vi "Autonomous Independent.vi"() -> ()   [LabVIEW 2013]
doc: "This VI is called when autonomous begins, and will automatically be terminated when autonomous ends. You can carry out timed or sensor driven robot movement independently without needing to return to the caller."
uses:
  Program Files (x86)/National Instruments/LabVIEW 2013/examples/FRC/I2C/ADXL345 I2C/Driver/ADXL345 I2C Axis.ctl
  Robot Global Data.vi
  <vilib>/addons/control/pid/pid.llb/PID (DBL).vi
  <vilib>/Rock Robotics/WPI/RobotDrive/WPI_RobotDriveGetSetRefNum.vi
  <vilib>/Rock Robotics/WPI/Joystick/WPI_JoystickGetSetRefNum.vi
  <vilib>/Rock Robotics/WPI/RobotDrive/WPI_RobotDriveArcadeDrive_Standard(NoSaturation).vi
  <vilib>/addons/control/pid/NI_PID_pid.lvlib
panel:
  in  "PID gains":T1={"proportional gain (Kc)"=1.0, "integral time (Ti, min)"=0.01, "derivative time (Td, min)"=0.0} {"derivative time (Td, min)" format="%.3f"; "integral time (Ti, min)" format="%.3f"; "proportional gain (Kc)" format="%.3f"}
  in  "Stop":bool
  in  "SP:":dbl(slide)=60.7843137254902 min=0.0 max=0.0 scale=0.0..100.0
  out "MV:":dbl(slide)=18.78965245852964 scale=-100.0..100.0
  out "Current Movement, for debugging":T2 {"Y Joystick Value" scale=1.0..-1.0; "X Joystick Value" scale=-1.0..1.0}
  in  "Array of robot movements":T3(array[cluster]) {"Y Joystick Value" scale=1.0..-1.0; "X Joystick Value" scale=-1.0..1.0}
  # "Be sure to right-click and choose Data Operations>>Make Current Value default if you want to save the array values with the VI"
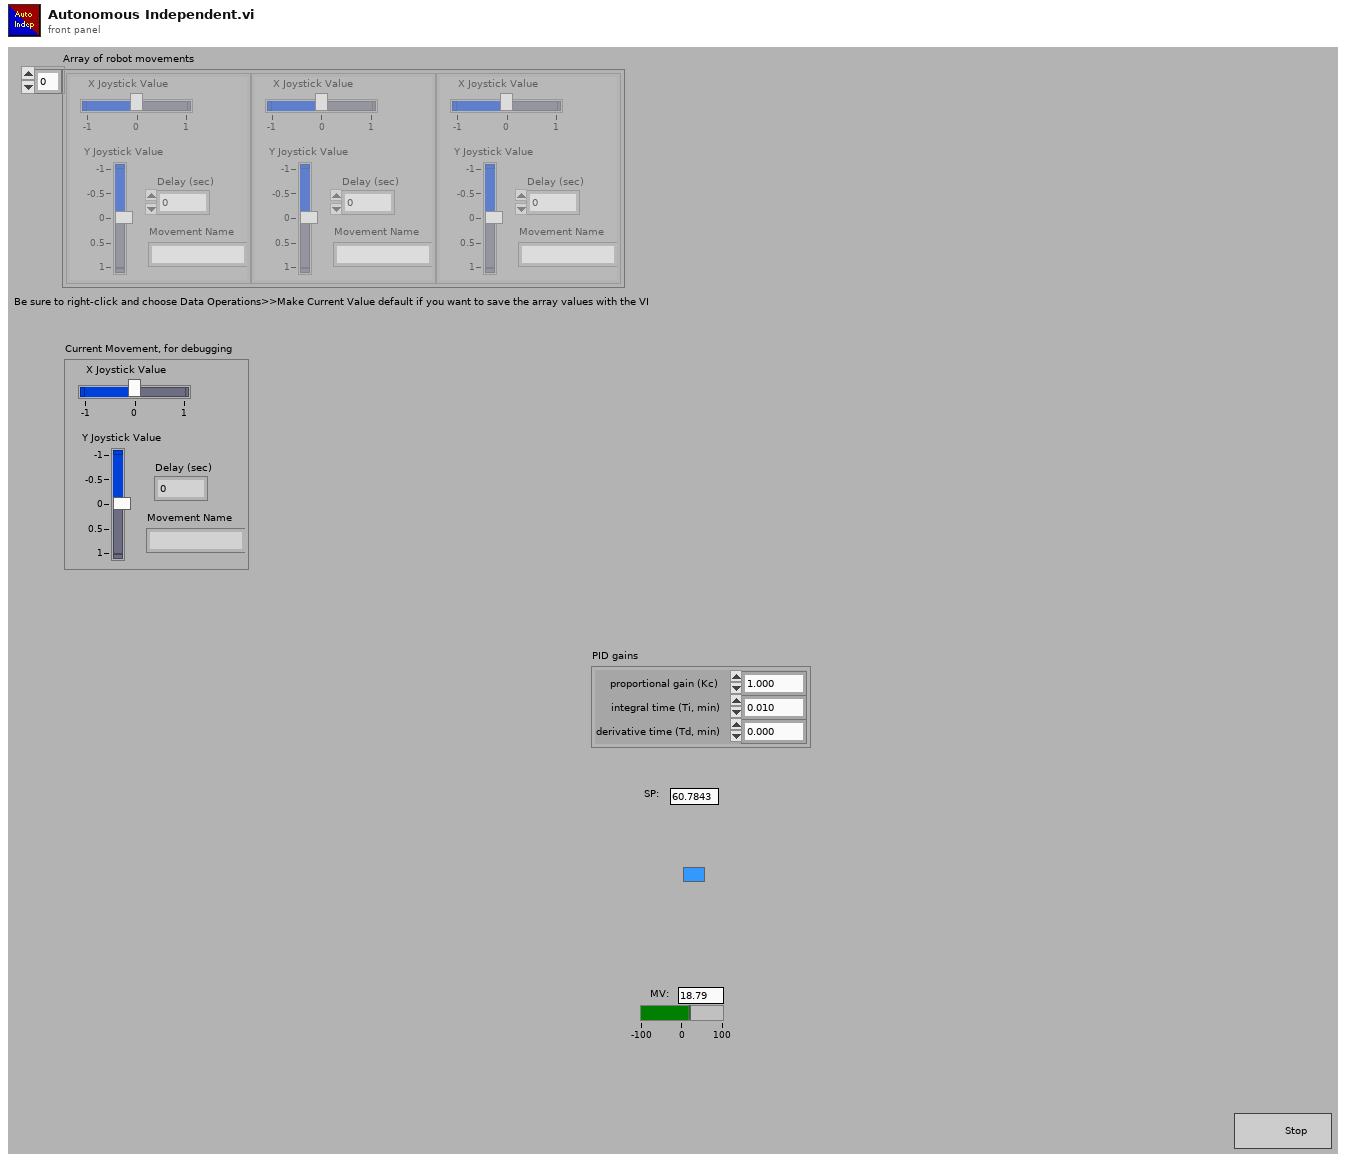
[diagram p1: front panel]
types:
  T1 = cluster{"proportional gain (Kc)":dbl, "integral time (Ti, min)":dbl, "derivative time (Td, min)":dbl}
  T2 = cluster{"X Joystick Value":dbl, "Y Joystick Value":dbl, "Delay (sec)":dbl, "Movement Name":string}
  T3 = cluster{"X Joystick Value":dbl, "Y Joystick Value":dbl, "Delay (sec)":dbl, "Movement Name":string}[]
  T4 = typedef "WPI_JoystickDevRef.ctl" = cluster{"Device":T5}
  T5 = typedef "WPI_JoystickDeviceEnum.ctl" = enum16{"USB 1", "USB 2", "USB 3", "USB 4", "Kinect 1", "Kinect 2"}
  T6 = typedef "WPI_EncoderDevRef.ctl" = cluster{"DevStatus":errorcluster, "EncoderIndex":T7, "CounterIndex":T8, "DistancePerCount":dbl, "Decoding Type":T9}
  T7 = typedef "FPGA_EncoderIdx.ctl" = enum8{"Enc 0", "Enc 1", "Enc 2", "Enc 3", "Invalid"}
  T8 = typedef "FPGA_CounterCtrSystemIndex.ctl" = enum8{"Ctr 0", "Ctr 1", "Ctr 2", "Ctr 3", "Ctr 4", "Ctr 5", "Ctr 6", "Ctr 7", "Invalid"}
  T9 = typedef "WPI_EncoderType.ctl" = enum16{"1x", "2x", "4x"}
  T10 = cluster{"axis 1 (x)":dbl, "axis 2 (y)":dbl, "axis 3 (throttle)":dbl, "axis 4":dbl, "axis 5":dbl, "axis 6":dbl}
  T11 = typedef "WPI_I2CDevRef.ctl" = cluster{"DevStatus":errorcluster, "Digital Module":T12, "Device Address":u8}
  T12 = typedef "FPGA_TypedefDigitalModule.ctl" = enum16{"Digital Module 1", "Digital Module 2"}
  T13 = typedef "WPI_RobotDriveDevRef.ctl" = cluster{"DevStatus":errorcluster, "Motors[]":T14[], "Square Inputs":bool, "Max Output":dbl, "Isochronous":bool}
  T14 = typedef "WPI_MotorControlDeviceRef.ctl" = cluster{"DeviceStatus":errorcluster, "Type":enum16{"PWM", "CAN"}, "PWM":cluster{"Digital Module":T12, "PWM Channel":T15, "DeadBand":T16}, "CAN":cluster{"Device Number":u8, "Control Mode":T17, "Semaphore":T18, "Max Vout":dbl}, "Invert":bool, "TransformRef":T19, "InvTransformRef":T19}
  T15 = typedef "FPGA_DIOPWMChannel.ctl" = enum8{"PWM 1", "PWM 2", "PWM 3", "PWM 4", "PWM 5", "PWM 6", "PWM 7", "PWM 8", "PWM 9", "PWM 10", "Invalid"}
  T16 = typedef "WPI_PWMDeadband.ctl" = cluster{"Name":string, "maxPositivePwm":i32, "minPositivePwm":i32, "centerPwm":i32, "maxNegativePwm":i32, "minNegativePwm":i32, "angularRange":u16}
  T17 = typedef "WPI_CANJaguar_ControlMode.ctl" = enum8{"Percent VBus", "Current", "Speed", "Position", "Voltage"}
  T18 = typedef "Semaphore RefNum" = refnum<k1>
  T19 = typedef "WPI_PWMTransform_ConPane.ctl" = refnum<vi>
  T20 = typedef "ADXL345 I2C Axis.ctl" = u8
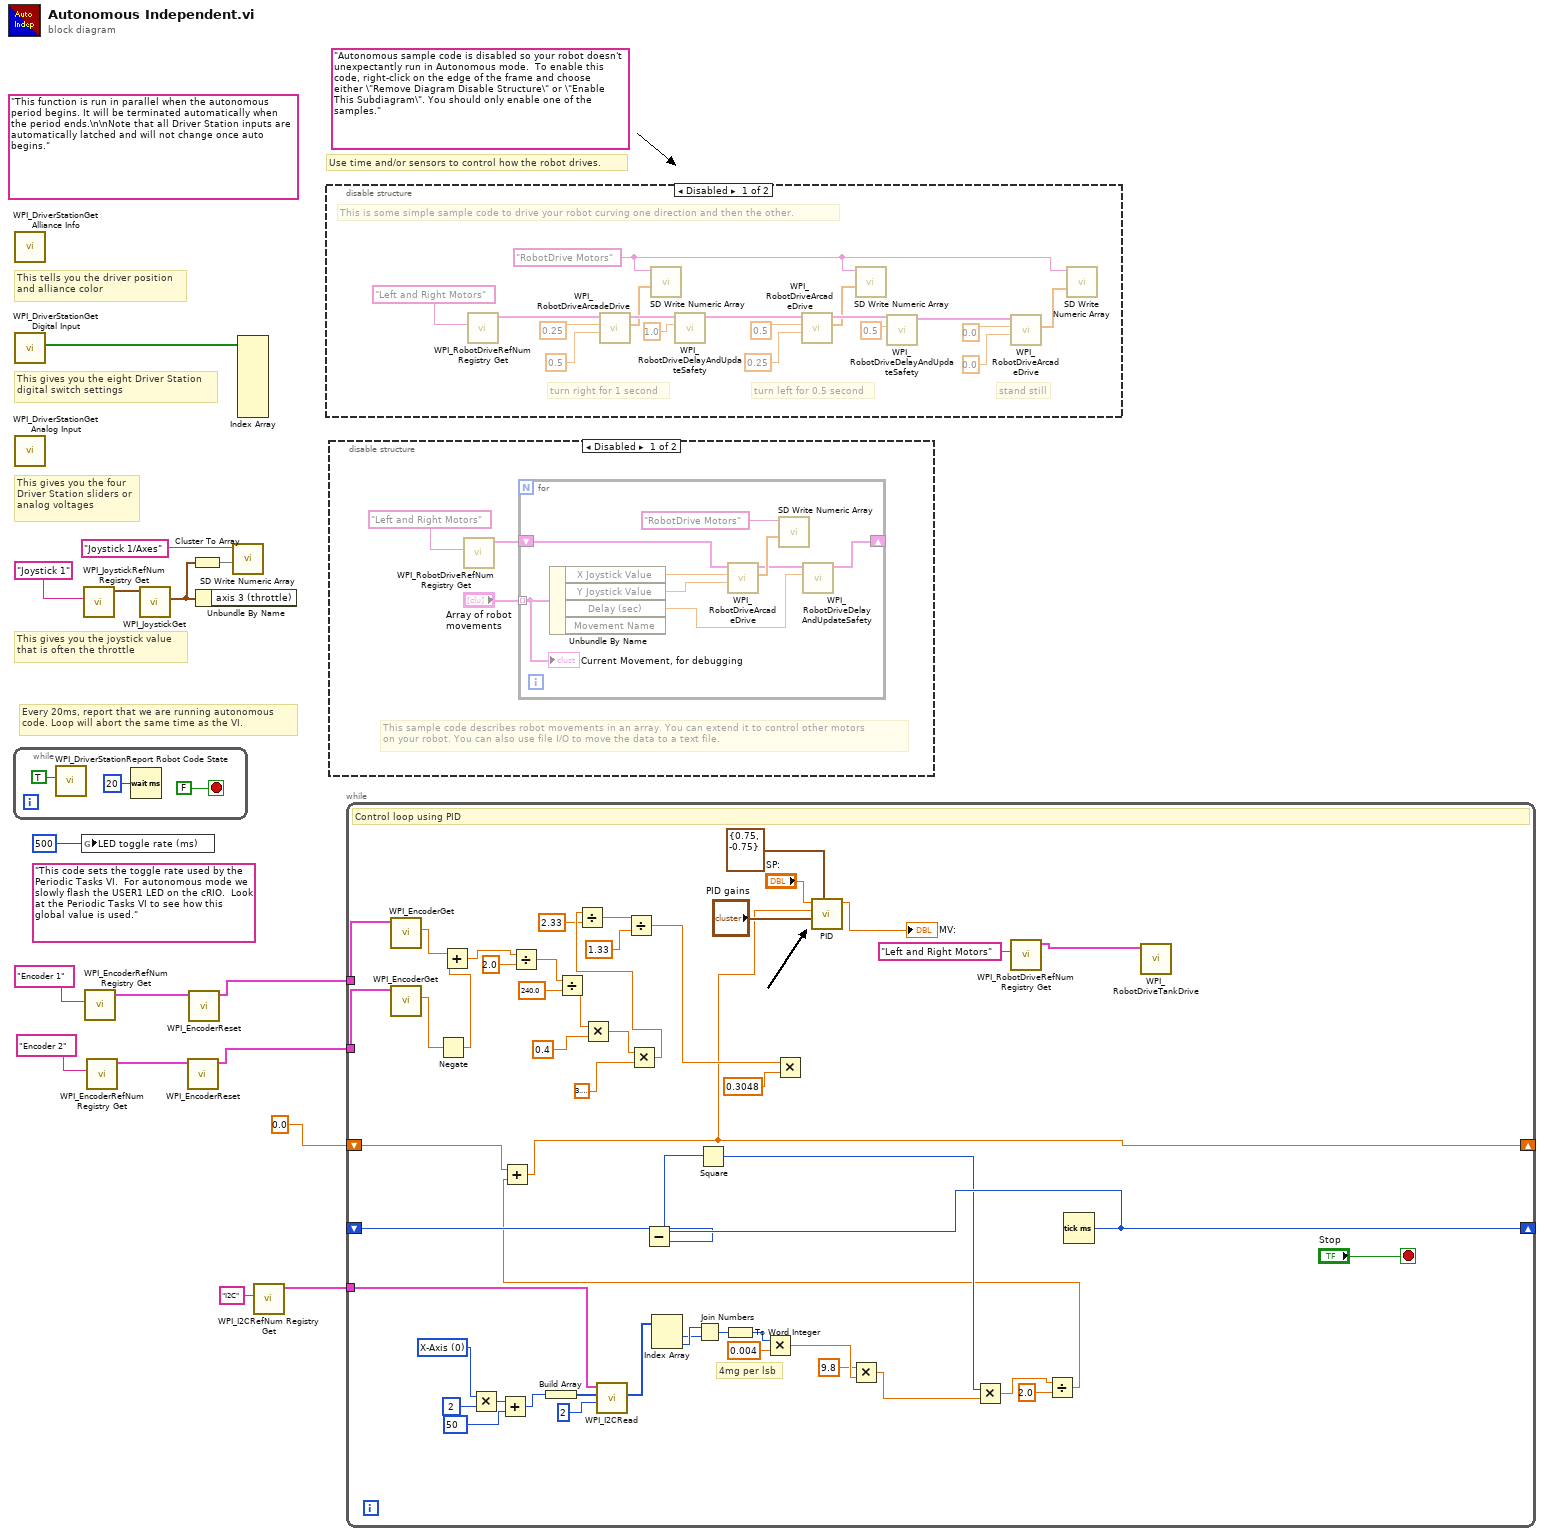
[diagram p0: block diagram]
diagram:
  (unwired) "This code sets the toggle rate used by the Periodic Tasks VI.  For autonomous mode we slowly flash the USER1 LED on the cRIO.  Look at the Periodic Tasks VI to see how this global value is used."
  (unwired) "Autonomous sample code is disabled so your robot doesn't unexpectantly run in Autonomous mode.  To enable this code, right-click on the edge of the frame and choose either \"Remove Diagram Disable Structure\" or \"Enable This Subdiagram\". You should only enable one of the samples."
  (unwired) "This function is run in parallel when the autonomous period begins. It will be terminated automatically when the period ends.\n\nNote that all Driver Station inputs are automatically latched and will not change once auto begins."
  # "Every 20ms, report that we are running autonomous\ncode. Loop will abort the same time as the VI."
  # "This gives you the joystick value\nthat is often the throttle"
  # "Use time and/or sensors to control how the robot drives."
  # "This tells you the driver position\nand alliance color"
  # "This gives you the eight Driver Station\ndigital switch settings"
  # "This gives you the four\nDriver Station sliders or\nanalog voltages"
  n1 = while {
    stop <- FALSE stop-if-true
    n2 = call <vilib>:"WPI_DriverStationReport Robot Code State.vi"("Autonomous"=TRUE) -> ()  [unwired: 10 in, 1 out]
    n3 = Wait (ms)(milliseconds to wait=u32 20) -> ()  [unwired: 1 out]
  }
  n4 = call <vilib>:"WPI_DriverStationGet Alliance Info.vi"() -> ()  [unwired: 12 out]
  n5 = call <vilib>:"WPI_DriverStationGet Digital Input.vi"() -> ("Driver Station Digital Input (1-8)"=w16:bool[])  [unwired: 11 out]
  n6 = call <vilib>:"WPI_DriverStationGet Analog Input.vi"() -> ()  [unwired: 12 out]
  n7 = global write "Robot Global Data.vi" "LED toggle rate (ms)"(u32 500 ("LED ms toggle rate")) -> ()
  n8 = call <vilib>:"WPI_JoystickRefNum Registry Get.vi"("refnum name"="Joystick 1") -> ("JoystickDevRef"=w14:T4)  [unwired: 1 in, 9 out]
  n9 = call <vilib>:"WPI_EncoderRefNum Registry Get.vi"("refnum name"="Encoder 1") -> ("EncoderDevRef"=w6:T6)  [unwired: 9 in, 1 out]
  n10 = call <vilib>:"WPI_EncoderRefNum Registry Get.vi"("refnum name"="Encoder 2") -> ("EncoderDevRef"=w7:T6)  [unwired: 9 in, 1 out]
  n11 = call <vilib>:"WPI_JoystickGet.vi"("JoystickDevRef"=w14) -> ("Axes"=w11:T10)  [unwired: 1 in, 5 out]
  n12 = call <vilib>:"WPI_EncoderReset.vi"("EncoderDevRef"=w7) -> ("EncoderDevRef"=w4:T6)  [unwired: 9 in, 1 out]
  n13 = call <vilib>:"WPI_EncoderReset.vi"("EncoderDevRef"=w6) -> ("EncoderDevRef"=w5:T6)  [unwired: 9 in, 1 out]
  n14 = Cluster To Array(cluster=w11) -> (array=w12:dbl[])
  n15 = Unbundle By Name(w11) -> ()  [unwired: 1 out]
  n16 = call <vilib>:"SD Write Numeric Array.vi"("Numeric Array"=w12, "Name"="Joystick 1/Axes") -> ()  [unwired: 8 in, 2 out]
  n17 = Index Array(array=w16) -> ()  [unwired: 8 in, 8 out]
  n18 = call <vilib>:"WPI_I2CRefNum Registry Get.vi"("refnum name"="I2C") -> ("I2CDevRef"=w1:T11)  [unwired: 9 in, 1 out]
  n19 = disable-structure shown="Disabled" {
    frame Disabled {
      w20 = "RobotDrive Motors" ("Name")
      # "This is some simple sample code to drive your robot curving one direction and then the other."
      # "stand still"
      # "turn left for 0.5 second"
      # "turn right for 1 second"
      n20 = call <vilib>:"WPI_RobotDriveRefNum Registry Get.vi"("refnum name"="Left and Right Motors") -> ("RobotDriveDevRef"=w24:T13)  [unwired: 1 in, 9 out]
      n21 = call-poly <vilib>:"WPI_RobotDriveArcadeDrive.vi"("Y axis value"=0.5 ("X axis value"), "X axis value"=0.25, "RobotDriveDevRef"=w24) -> ("Motor Values"=w23:dbl[], "RobotDriveDevRef"=w31:T13)  [unwired: 1 in, 6 out]
      n22 = call <vilib>:"SD Write Numeric Array.vi"("Numeric Array"=w23, "Name"=w20) -> ()  [unwired: 8 in, 2 out]
      n23 = call <vilib>:"WPI_RobotDriveDelayAndUpdateSafety.vi"("Delay (s)"=1.0, "RobotDriveDevRef"=w31) -> ("RobotDriveDevRef 2"=w30:T13)  [unwired: 8 in, 1 out]
      n24 = call-poly <vilib>:"WPI_RobotDriveArcadeDrive.vi"("Y axis value"=0.25 ("X axis value"), "X axis value"=0.5, "RobotDriveDevRef"=w30) -> ("Motor Values"=w22:dbl[], "RobotDriveDevRef"=w29:T13)  [unwired: 1 in, 6 out]
      n25 = call <vilib>:"SD Write Numeric Array.vi"("Numeric Array"=w22, "Name"=w20) -> ()  [unwired: 8 in, 2 out]
      n26 = call <vilib>:"WPI_RobotDriveDelayAndUpdateSafety.vi"("Delay (s)"=0.5, "RobotDriveDevRef"=w29) -> ("RobotDriveDevRef 2"=w28:T13)  [unwired: 8 in, 1 out]
      n27 = call-poly <vilib>:"WPI_RobotDriveArcadeDrive.vi"("Y axis value"=0.0 ("X axis value"), "X axis value"=0.0, "RobotDriveDevRef"=w28) -> ("Motor Values"=w21:dbl[])  [unwired: 1 in, 7 out]
      n28 = call <vilib>:"SD Write Numeric Array.vi"("Numeric Array"=w21, "Name"=w20) -> ()  [unwired: 8 in, 2 out]
    }
    frame Enabled {
    }
  }
  n29 = disable-structure shown="Disabled" {
    frame Disabled {
      # "This sample code describes robot movements in an array. You can extend it to control other motors\non your robot. You can also use file I/O to move the data to a text file."
      n30 = call <vilib>:"WPI_RobotDriveRefNum Registry Get.vi"("refnum name"="Left and Right Motors") -> ("RobotDriveDevRef"=w39:T13)  [unwired: 1 in, 9 out]
      n31 = for {
        shift-right: [w45] -> _
        shift-left: w39 -> [w46]
        tunnel: "Array of robot movements" -> [w41] mode=indexing
        n32 = Unbundle By Name(w41) -> ("X Joystick Value"=w44:dbl, "Y Joystick Value"=w43:dbl, "Delay (sec)"=w42:dbl)  [unwired: 1 out]
        n33 = call-poly <vilib>:"WPI_RobotDriveArcadeDrive.vi"("Y axis value"=w43, "X axis value"=w44, "RobotDriveDevRef"=w46) -> ("Motor Values"=w48:dbl[], "RobotDriveDevRef"=w47:T13)  [unwired: 1 in, 6 out]
        n34 = call <vilib>:"SD Write Numeric Array.vi"("Numeric Array"=w48, "Name"="RobotDrive Motors") -> ()  [unwired: 8 in, 2 out]
        n35 = call <vilib>:"WPI_RobotDriveDelayAndUpdateSafety.vi"("Delay (s)"=w42, "RobotDriveDevRef"=w47) -> ("RobotDriveDevRef 2"=w45:T13)  [unwired: 8 in, 1 out]
        "Current Movement, for debugging" <- w41
      }
    }
    frame Enabled {
    }
  }
  n36 = while {
    tunnel: w5 -> [w99]
    tunnel: w4 -> [w98]
    shift-right: [w76] -> _
    shift-left: _ -> [w75]
    shift-right: [w50] -> _
    shift-left: 0.0 -> [w77]
    tunnel: w1 -> [w60]
    stop <- "Stop" stop-if-true
    w72 = T20 0 items=["X-Axis", "Y-Axis", "Z-Axis"] ("Axis")
    # "4mg per lsb"
    # "Control loop using PID"
    n37 = call <vilib>:"WPI_EncoderGet.vi"("EncoderDevRef"=w99) -> ("Distance"=w97:dbl)  [unwired: 5 in, 5 out]
    n38 = call <vilib>:"WPI_EncoderGet.vi"("EncoderDevRef"=w98) -> ("Distance"=w84:dbl)  [unwired: 5 in, 5 out]
    n39 = Negate(x=w84) -> (-x=w83:dbl)
    n40 = Add(x=w97, y=w83) -> (x+y=w95:dbl)
    n41 = Multiply(x=w72, y=u8 2 ("Data To Send")) -> (x*y=w61:T20)
    n42 = Add(x=w61, y=u8 50 ("Data To Send")) -> (x+y=w69:T20)
    n43 = Divide(x=w95, y=2.0) -> (x/y=w85:dbl)
    n44 = Build Array(w69) -> (w70:T20[])
    n45 = Divide(x=w85, y=240.0) -> (x/y=w93:dbl)
    n46 = Multiply(x=w93, y=0.4) -> (x*y=w90:dbl)
    n47 = call <vilib>:"WPI_I2CRead.vi"("I2CBytesToRead"=u8 2, "I2CRegister"=w70, "I2CDevRef"=w60) -> ("Data Out"=w65:u8[])  [unwired: 2 in, 6 out]
    n48 = Multiply(x=w90, y=3.141592653589793) -> (x*y=w82:dbl)
    n49 = Divide(x=w82, y=2.33) -> (x/y=w80:dbl)
    n50 = Divide(x=w80, y=1.33) -> (x/y=w57:dbl)
    n51 = Index Array(array=w65) -> (element #1=w67:u8, element #2=w68:u8)  [unwired: 2 in]
    n52 = Join Numbers(hi=w68, lo=w67) -> ((hi.lo)=w66:u16)
    n53 = To Word Integer(number=w66) -> (16bit integer=w73:i16)
    n54 = Multiply(x=w73, y=0.004) -> (x*y=w59:dbl)
    n55 = Multiply(x=w57, y=0.3048) -> ()  [unwired: 1 out]
    n56 = Multiply(x=9.8, y=w59) -> (x*y=w54:dbl)
    n57 = call <vilib>:"WPI_RobotDriveRefNum Registry Get.vi"("refnum name"="Left and Right Motors") -> ("RobotDriveDevRef"=w86:T13)  [unwired: 9 in, 1 out]
    n58 = Tick Count (ms)() -> (millisecond timer value=w76:u32)
    n59 = Subtract(x=w76, y=w75) -> (x-y=w74:u32)
    n60 = Square(x=w74) -> (x^2=w55:u32)
    n61 = Multiply(x=w55, y=w54) -> (x*y=w52:dbl)
    n62 = Divide(x=w52, y=2.0) -> (x/y=w51:dbl)
    n63 = Add(x=w77, y=w51) -> (x+y=w50:dbl)
    n64 = call-poly <vilib>:"PID.vi"("output range"=cluster{"output high":dbl, "output low":dbl} {"output high"=0.75, "output low"=-0.75}, "PID gains"="PID gains", "process variable"=w50, "setpoint"="SP:") -> ("output"=→"MV:":dbl)  [unwired: 6 in, 1 out]
    n65 = call <vilib>:"WPI_RobotDriveTankDrive.vi"("RobotDriveDevRef"=w86) -> ()  [unwired: 8 in, 3 out]
  }
